vi "Send station config update event.vi"(8 "error in (no error)":errorcluster, 11 "Station config in":refnum<class "Station config.lvclass">) -> (0 "error out":errorcluster, 3 "Station config out":refnum<class "Station config.lvclass">)   [LabVIEW 2018]
doc: "This sends an event sending the Station Config data passed in to the Model case of the main VI. This event should be fired whenever the Station Config object in the main state loop updates to trigger an update for any controls based on it."
uses:
  <userlib>/Recipe/Station Config/Station config.lvclass
  References/Fiber Auto Collimation References.lvclass
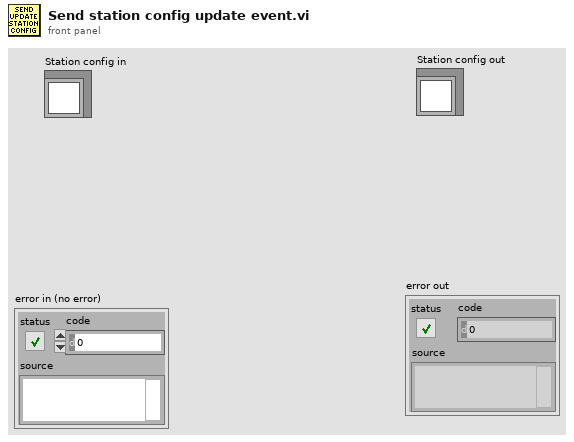
[diagram p1: front panel]
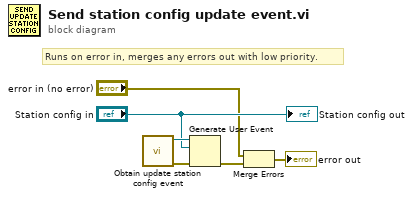
[diagram p0: block diagram]
diagram:
  # "Runs on error in, merges any errors out with low priority."
  n1 = call "Obtain update station config event.vi"() -> ("error out"=w6:errorcluster, "Update Station config"=w5:refnum<user-event>)  [unwired: 10 in]
  n2 = Generate User Event(user event=w5, event data cluster="Station config in", error in=w6) -> (error out=w3:errorcluster)  [unwired: 1 in, 1 out]
  n3 = Merge Errors("error in (no error)", w3) -> (→"error out":errorcluster)
  "Station config out" <- "Station config in"
